vi "Initialise Zap Sat.vi"(8 "error in (no error)":errorcluster, 10 "Renderer":u32, 11 "Deployable in":refnum<class "Zap Sat.lvclass">) -> (0 "error out":errorcluster, 3 "Deployable out":refnum<class "Zap Sat.lvclass">)   [LabVIEW 2021, in "Zap Sat.lvclass"]
uses:
  Zap Sat.lvclass
  Zap Sat.lvclass/Zap Sat.ctl
  C:/dev/LabVIEW/LabMelee/Source/Application Specific/Deployable/Deployable.lvclass
  C:/dev/LabVIEW/LabMelee/Source/Application Specific/Element/Element.lvclass
  C:/dev/LabVIEW/LabMelee/Source/Application Specific/Deployables/Zap Sat/Zap Sat.lvclass
  Deployable/Deployable.lvclass
  Actors/Main Controller/Actor/Player.ctl
  Actors/Main Controller/Actor/Main Controller Actor.lvclass
panel:
  in  "Owner":T1
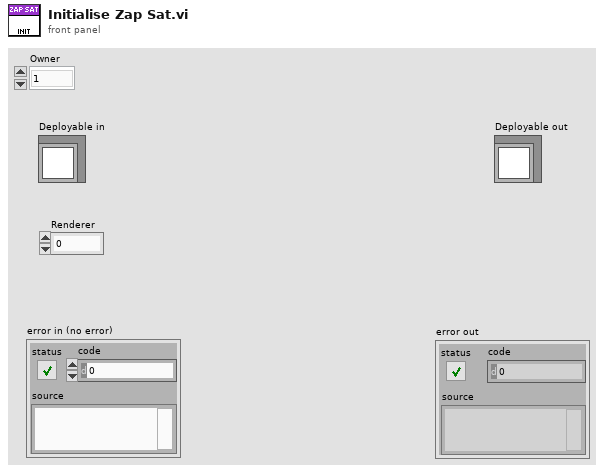
[diagram p1: front panel]
types:
  T1 = typedef "Main Controller Actor.lvclass/Player.ctl" = enum16{"1", "2"}
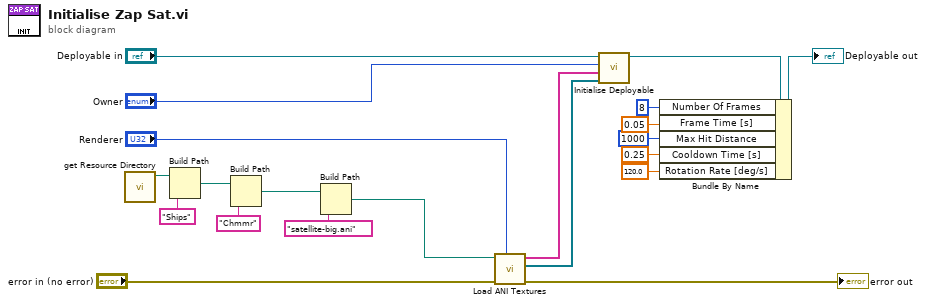
[diagram p0: block diagram]
diagram:
  n1 = call "get Resource Directory.vi"() -> ("Resource Directory"=w17:path)  [unwired: 11 in]
  n2 = Build Path(base path=w17, name or relative path="Ships") -> (appended path=w15:path)
  n3 = Build Path(base path=w15, name or relative path="Chmmr") -> (appended path=w19:path)
  n4 = Build Path(base path=w19, name or relative path="satellite-big.ani" ("format string")) -> (appended path=w14:path)
  n5 = call "Load ANI Textures.vi"("Renderer"="Renderer", "error in (no error)"="error in (no error)", "Path"=w14) -> ("error out"=→"error out":errorcluster, "Hotspots"=w6:refnum<class "Vector 2D.lvclass">[], "Names"=w7:string[])  [unwired: 6 in]
  n6 = call "Initialise Deployable.vi"("Hotspots"=w6, "Textures"=w7, "Owner"="Owner", "Deployable in"="Deployable in") -> ("Deployable out"=w10:refnum<class "Zap Sat.lvclass">)  [unwired: 7 in]
  n7 = Bundle By Name(cluster=w10, "Number Of Frames"=8, "Frame Time [s]"=0.05, "Max Hit Distance"=1000, "Cooldown Time [s]"=0.25, "Rotation Rate [deg/s]"=sgl 120.0) -> (→"Deployable out":refnum<class "Zap Sat.lvclass">)
